vi "GetParam.vi"(8 "error in (no error)":errorcluster caption="entrée d'erreur (pas d'erreur)", 11 "RepeatedStratifiedKFold.lvclass":refnum<class "RepeatedStratifiedKFold.lvclass">) -> (0 "error out":errorcluster caption="sortie d'erreur", 2 "RepeatedStratifiedKFold":T1={"n_splits"=5, "n_repeats"=10, "random_state"=-1} {"random_state" min=-1}, 3 "RepeatedStratifiedKFold.lvclass":refnum<class "RepeatedStratifiedKFold.lvclass">)   [LabVIEW 2020, in "RepeatedStratifiedKFold.lvclass"]
doc: "Get Parameters"
uses:
  RepeatedStratifiedKFold.lvclass
  RepeatedStratifiedKFold.lvclass/RepeatedStratifiedKFold.ctl
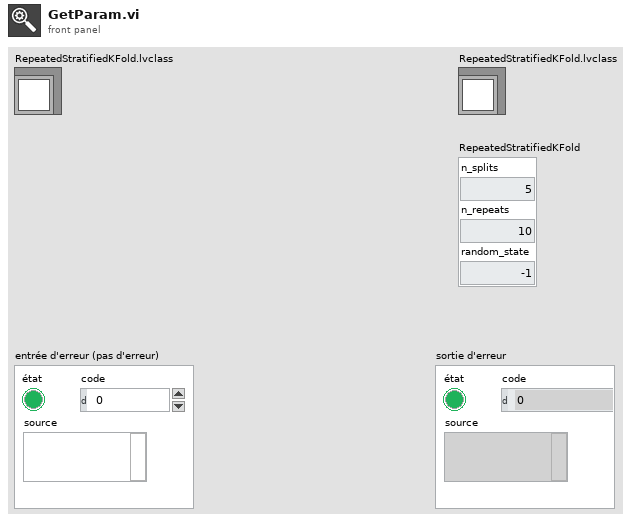
[diagram p1: front panel]
types:
  T1 = cluster{"n_splits":i32, "n_repeats":i32, "random_state":i32}
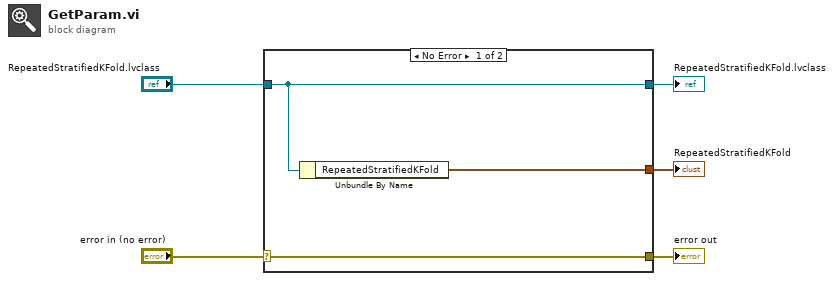
[diagram p0: block diagram]
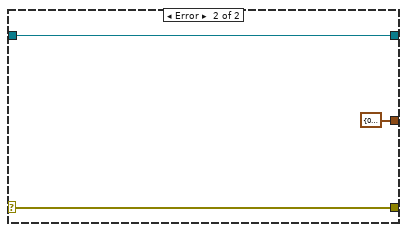
[diagram p2: hidden frame]
diagram:
  n1 = case shown="No Error" "error in (no error)" {
    selector: "error in (no error)" -> [w8 w10]
    tunnel: [w8 w10] -> w4
    tunnel: [w7 w11] -> w2
    tunnel: "RepeatedStratifiedKFold.lvclass" -> [w7 w11]
    tunnel: [w6 T1 {"n_splits"=0, "n_repeats"=0, "random_state"=0} ("RepeatedStratifiedKFold")] -> w1
    frame No Error {
      n2 = Unbundle By Name(w7) -> ("RepeatedStratifiedKFold"=w6:T1)
    }
    frame Error {
    }
  }
  "error out" <- w4
  "RepeatedStratifiedKFold.lvclass" <- w2
  "RepeatedStratifiedKFold" <- w1
